vi "CRC计算.vi"(1 "无校验U8数组":u8[](array[numeric])) -> (14 "计算后字符串":string, 16 "CRC值":u16)   [LabVIEW 2019]
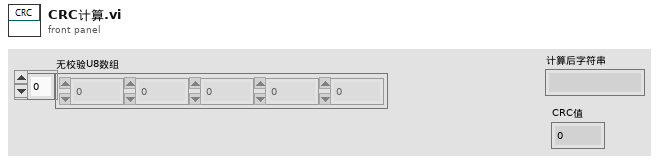
[diagram p1: front panel]
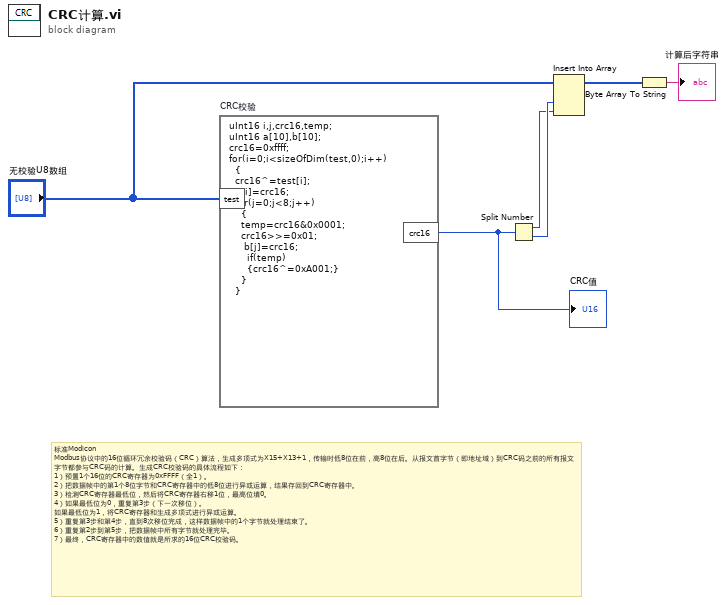
[diagram p0: block diagram]
diagram:
  # "标准Modicon Modbus协议中的16位循环冗余校验码（CRC）算法，生成多项式为X15+X13+1，传输时低8位在前，高8位在后。从报文首字节（即地址域）到CRC码之前的所有报文字节都参与CRC码的计算。生成CRC校验码的具体流程如下：\n1）预置1个16位的CRC寄存器为0xFFFF（全1）。\n2）把数据帧中的第1个8位字节和CRC寄存器中的低8位进行异或运算，结果存回到CRC寄存器中。\n3）检测CRC寄存器最低位，然后将CRC寄存器右移1位，最高位填0。\n4）如果最低位为0，重复第3步（下一次移位）。\n如果最低位为1，将CRC寄存器和生成多项式进行异或运算。\n5）重复第3步和第4步，直到8次移位完成，这样数据帧中的1个字节就处理结束了。\n6）重复第2步到第5步，把数据帧中所有字节就处理完毕。\n7）最终，CRC寄存器中的数值就是所求的16位CRC校验码。"
  n1 = formula code="uInt16 i,j,crc16,temp;\nuInt16 a[10],b[10];\ncrc16=0xffff;\nfor(i=0;i<sizeOfDim(test,0);i++)\n  {\n  crc16^=test[i];\n  a[i]=crc16;\n  for(j=0;j<8;j++)\n    {\n    temp=crc16&0x0001;\n    crc16>>=0x01;\n     b[j]=crc16;\n      if(temp)\n      {crc16^=0xA001;}\n    }\n  }" "CRC校验"("test"="无校验U8数组") -> ("crc16"=w6:u16)
  "CRC值" <- w6
  n2 = Split Number(x=w6) -> (hi(x)=w1:u8, lo(x)=w2:u8)
  n3 = Insert Into Array(array="无校验U8数组", new element #1=w2, new element #2=w1) -> (w4:u8[])  [unwired: 1 in]
  n4 = Byte Array To String(unsigned byte array=w4) -> (string=→"计算后字符串":string)
